vi "chtotreeindex.vi"(10 "name":string[](array[string])) -> (2 "datatypeindex":T1[](array[typedef]))   [LabVIEW 2011]
uses:
  chdatatype.ctl
  config table enum.ctl
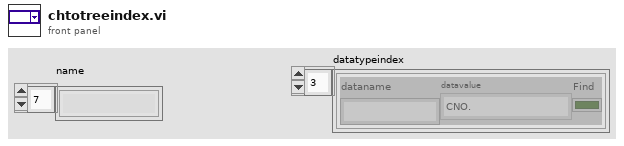
[diagram p1: front panel]
types:
  T1 = typedef "chdatatype.ctl" = cluster{"dataname":string, "datavalue":T2, "Find":bool}
  T2 = typedef "config table enum.ctl" = enum16{"CNO.", "CName", "CLASSI", "CLASSII", "ch", "Chname", "USE", "fre", "range", "senNO", "PHname", "unit", "CALclass", "K", "OFF", "Alrm", "filt", "Power", "display", "threshold", "compare", "Etype"}
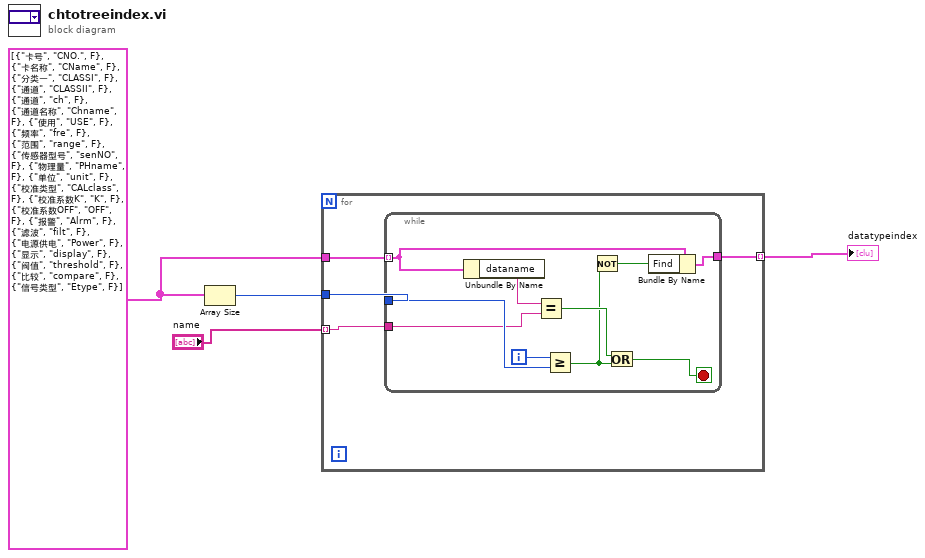
[diagram p0: block diagram]
diagram:
  w3 = T1[] [{"dataname"="卡号", "datavalue"=enum."CNO.", "Find"=FALSE}, {"dataname"="卡名称", "datavalue"=enum."CName", "Find"=FALSE}, {"dataname"="分类一", "datavalue"=enum."CLASSI", "Find"=FALSE}, {"dataname"="通道", "datavalue"=enum."CLASSII", "Find"=FALSE}, {"dataname"="通道", "datavalue"=enum."ch", "Find"=FALSE}, {"dataname"="通道名称", "datavalue"=enum."Chname", "Find"=FALSE}, {"dataname"="使用", "datavalue"=enum."USE", "Find"=FALSE}, {"dataname"="频率", "datavalue"=enum."fre", "Find"=FALSE}, {"dataname"="范围", "datavalue"=enum."range", "Find"=FALSE}, {"dataname"="传感器型号", "datavalue"=enum."senNO", "Find"=FALSE}, {"dataname"="物理量", "datavalue"=enum."PHname", "Find"=FALSE}, {"dataname"="单位", "datavalue"=enum."unit", "Find"=FALSE}, {"dataname"="校准类型", "datavalue"=enum."CALclass", "Find"=FALSE}, {"dataname"="校准系数K", "datavalue"=enum."K", "Find"=FALSE}, {"dataname"="校准系数OFF", "datavalue"=enum."OFF", "Find"=FALSE}, {"dataname"="报警", "datavalue"=enum."Alrm", "Find"=FALSE}, {"dataname"="滤波", "datavalue"=enum."filt", "Find"=FALSE}, {"dataname"="电源供电", "datavalue"=enum."Power", "Find"=FALSE}, {"dataname"="显示", "datavalue"=enum."display", "Find"=FALSE}, {"dataname"="阀值", "datavalue"=enum."threshold", "Find"=FALSE}, {"dataname"="比较", "datavalue"=enum."compare", "Find"=FALSE}, {"dataname"="信号类型", "datavalue"=enum."Etype", "Find"=FALSE}] ("Array")
  n1 = Array Size(array=w3) -> (size(s)=w2:i32)
  n2 = for {
    tunnel: "name" -> [w8] mode=indexing
    tunnel: w3 -> [w7]
    tunnel: w2 -> [w6]
    tunnel: [w5] -> w1 mode=indexing
    n3 = while {
      tunnel: w7 -> [w12] mode=indexing
      tunnel: w8 -> [w16]
      tunnel: w6 -> [w18]
      tunnel: [w10] -> w5
      i -> [w13]
      stop <- w14 stop-if-true
      n4 = Unbundle By Name(w12) -> ("dataname"=w17:string)
      n5 = Equal?(x=w17, y=w16) -> (x = y?=w15:bool)
      n6 = Greater Or Equal?(x=w13, y=w18) -> (x >= y?=w11:bool)
      n7 = Not(x=w11) -> (.not. x?=w9:bool)
      n8 = Or(x=w15, y=w11) -> (x .or. y?=w14:bool)
      n9 = Bundle By Name(cluster=w12, "Find"=w9) -> (w10:T1)
    }
  }
  "datatypeindex" <- w1
